vi "test-worker mode.vi"(8 "error in (no error)":errorcluster, 11 "TestCase in":refnum<class "testcase-CSMAttributes.lvclass">) -> (0 "error out":errorcluster, 3 "TestCase out":refnum<class "testcase-CSMAttributes.lvclass">)   [LabVIEW 2017, in "testcase-CSMAttributes.lvclass"]
uses:
  testcase-CSMAttributes.lvclass
  6faf3dd6-bbe3-43e6-ac0e-6a595a4bbb73.vi
  eea55257-98dc-4069-a2fc-7f3abec53d34.vi
  654a1434-e049-45b7-bbe1-b3daff27deed.vi
  232dea5e-886f-41b8-bb39-dacd9565842e.vi
  d39486ea-fbfe-4c2b-b0ae-85d31efdfc25.vi
  4fbfc3b2-4ab6-4b17-950e-362f3a1418f9.vi
  eb53d3db-f5cc-4d50-900d-3a282fe3921b.vi
  d3eb8ef0-7d19-473b-ace2-fe9805f10b86.vi
  src/user.lib/_NEVSTOP/Communicable State Machine(CSM)/AdvanceAPI/CSM - Set Module Attribute.vi
  src/user.lib/_NEVSTOP/Communicable State Machine(CSM)/AdvanceAPI/CSM - Get Module Attribute.vi
  src/user.lib/_NEVSTOP/Communicable State Machine(CSM)/Communicable State Machine.lvlib
  <vilib>/addons/_JKI Toolkits/VI Tester/TestCase.llb/TestCase.lvclass
  C:/Program Files (x86)/National Instruments/LabVIEW 2017/vi.lib/addons/_JKI Toolkits/VI Tester/TestCase.llb/TestCase.lvclass
panel:
  out "error out":errorcluster
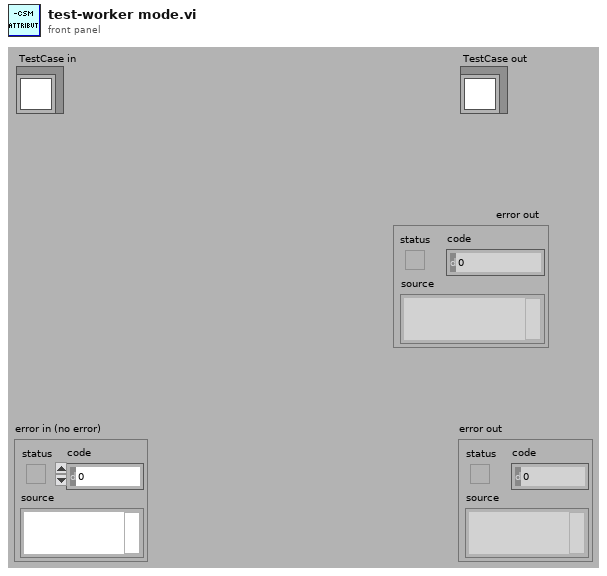
[diagram p1: front panel]
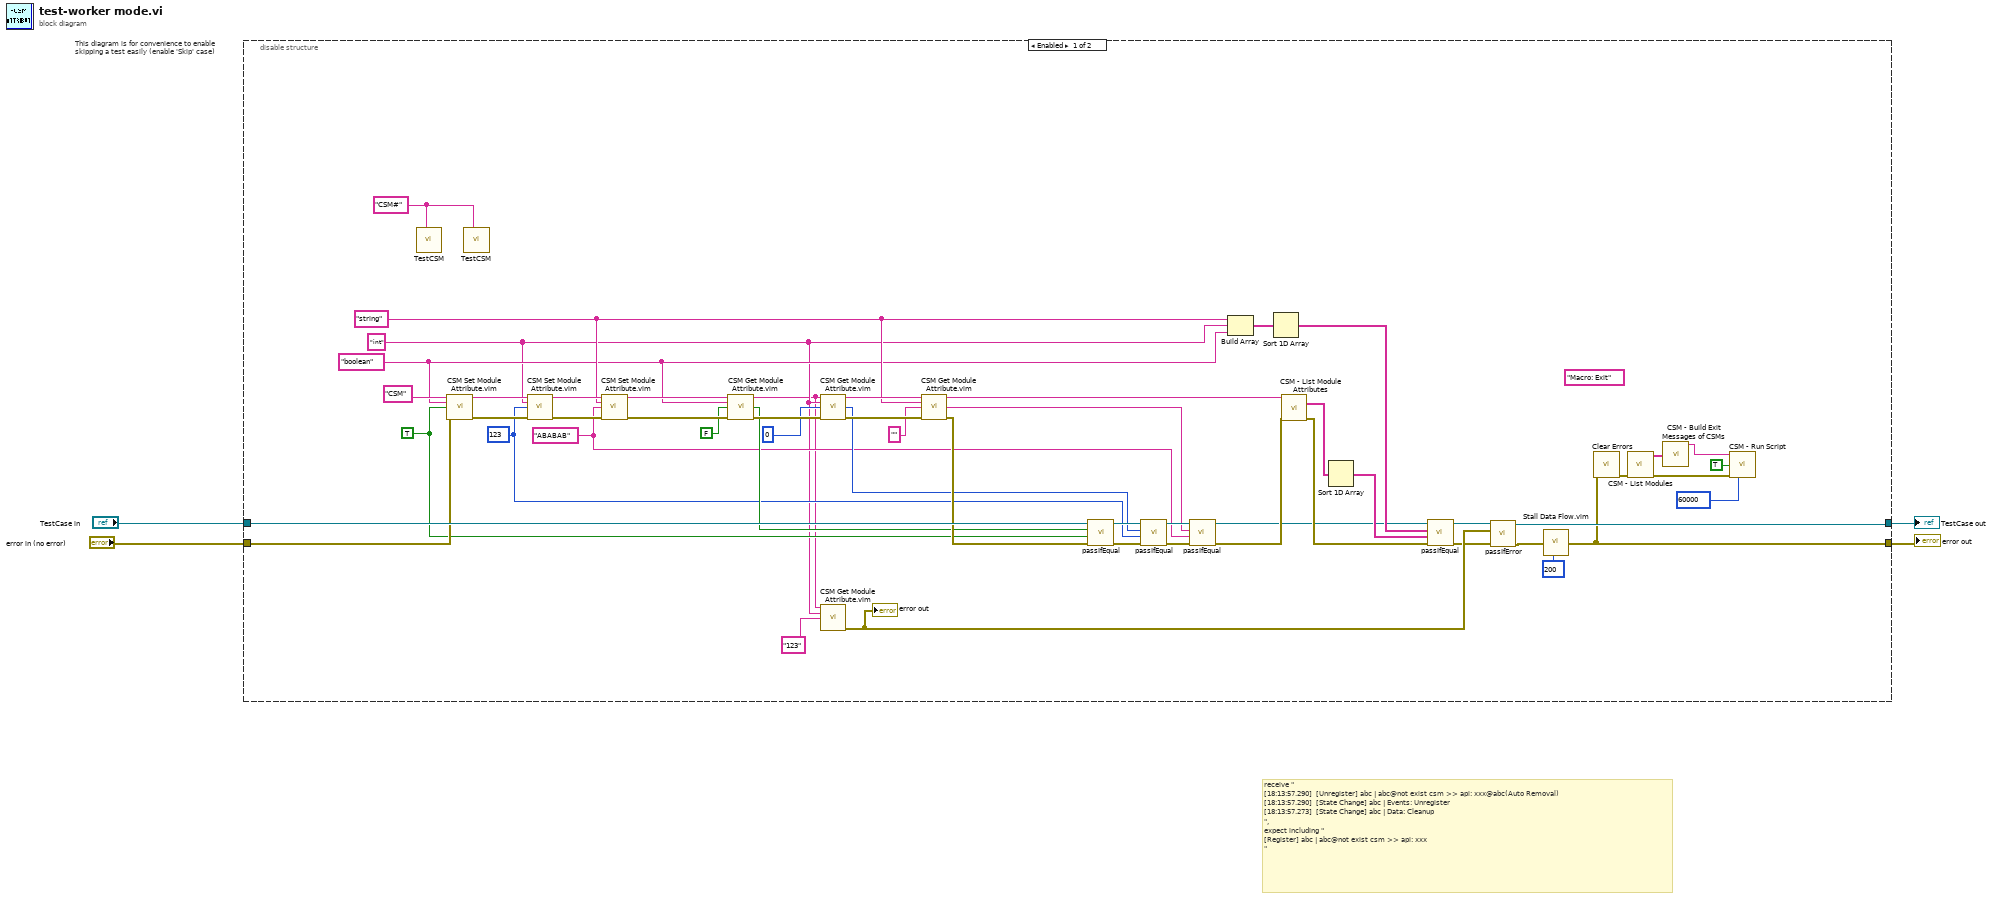
[diagram p0: block diagram]
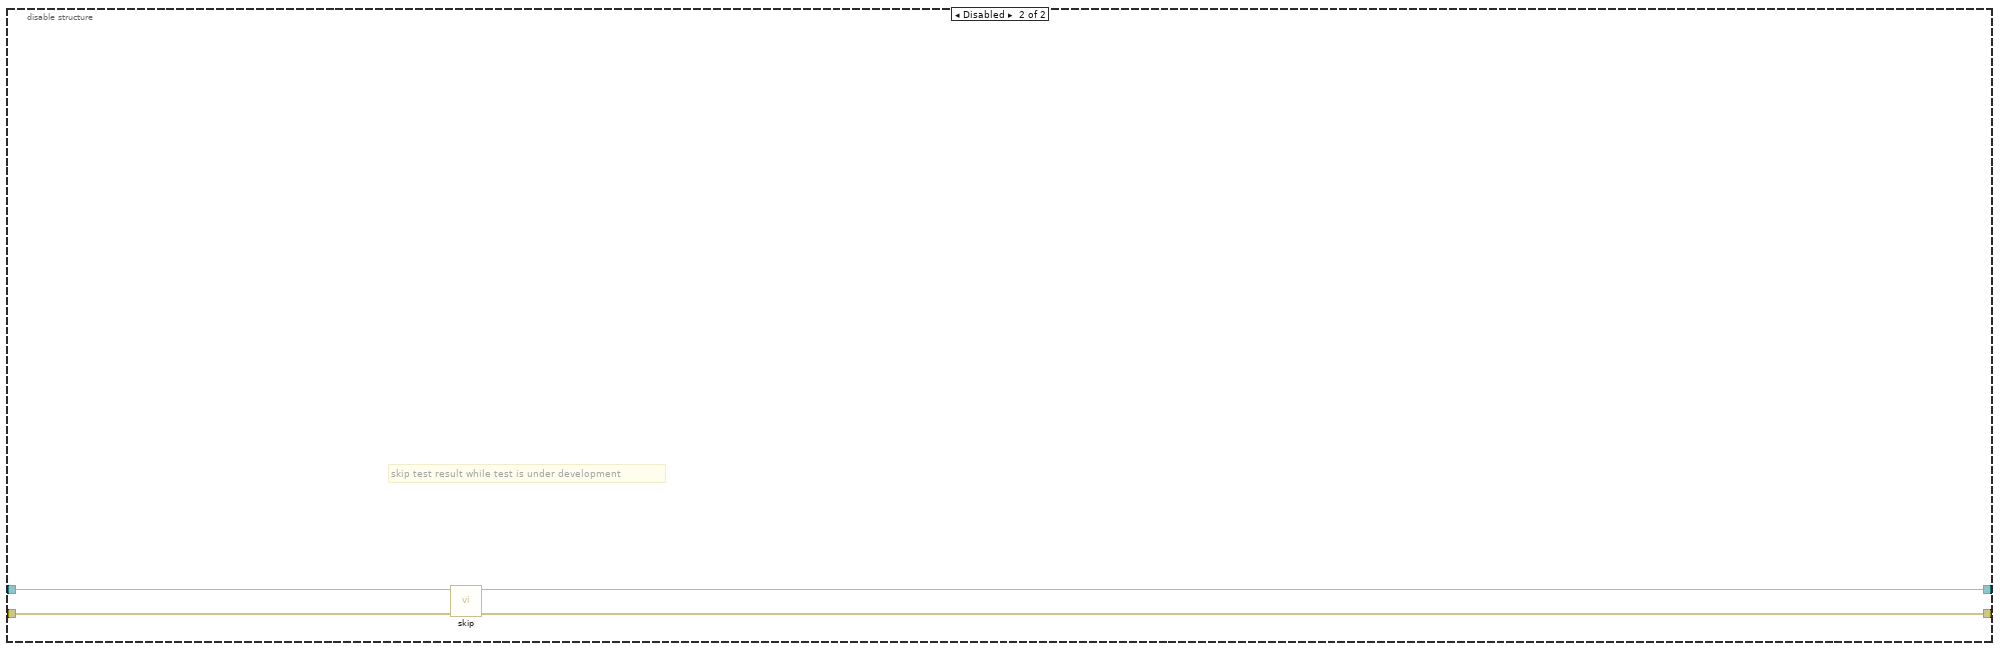
[diagram p2: hidden frame]
diagram:
  # "receive \"\n[18:13:57.290]  [Unregister] abc | abc@not exist csm >> api: xxx@abc(Auto Removal)\n[18:13:57.290]  [State Change] abc | Events: Unregister\n[18:13:57.273]  [State Change] abc | Data: Cleanup\n\", \nexpect including \"\n[Register] abc | abc@not exist csm >> api: xxx\n\""
  n1 = disable-structure "This diagram is for convenience to enable skipping a test easily (enable 'Skip' case)" shown="Enabled" {
    disable-tunnel: "TestCase in" -> [w57 w61]
    disable-tunnel: [w13 w59] -> w1
    disable-tunnel: [w7 w60] -> w3
    disable-tunnel: "error in (no error)" -> [w56 w58]
    frame Enabled {
      (unwired) "Macro: Exit" ("State")
      w32 = "ABABAB" ("Attribute")
      w28 = "string" ("Attribute")
      w36 = 123
      w19 = "int" ("Attribute")
      w41 = TRUE
      w27 = "boolean" ("Attribute")
      w12 = "CSM#" ("Name (\"\" to Use UUID)")
      n2 = call "TestCSM.vi"("Name (\"\" to Use UUID)"=w12) -> ()  [unwired: 11 in]
      n3 = call "CSM Set Module Attribute.vim"("CSM Name"="CSM" ("Name (\"\" to Use UUID)"), "Attribute"=w27, "Value"=w41, "Error In"=w56) -> ("CSM Name (Dup)"=w52:string, "error out"=w54:errorcluster)  [unwired: 8 in, 2 out]
      n4 = call "TestCSM.vi"("Name (\"\" to Use UUID)"=w12) -> ()  [unwired: 11 in]
      n5 = call "CSM Set Module Attribute.vim"("CSM Name"=w52, "Attribute"=w19, "Value"=w36, "Error In"=w54) -> ("CSM Name (Dup)"=w51:string, "error out"=w53:errorcluster)  [unwired: 8 in, 2 out]
      n6 = call "CSM Set Module Attribute.vim"("CSM Name"=w51, "Attribute"=w28, "Value"=w32, "Error In"=w53) -> ("CSM Name (Dup)"=w49:string, "error out"=w50:errorcluster)  [unwired: 8 in, 2 out]
      n7 = call "CSM Get Module Attribute.vim"("CSM Name"=w49, "Attribute"=w27, "Default Value (Empty Variant)"=FALSE, "Error In"=w50) -> ("CSM Name (Dup)"=w18:string, "Value"=w40:bool, "error out"=w48:errorcluster)  [unwired: 7 in, 2 out]
      n8 = call "CSM Get Module Attribute.vim"("CSM Name"=w18, "Attribute"=w19, "Default Value (Empty Variant)"=0, "Error In"=w48) -> ("CSM Name (Dup)"=w47:string, "Value"=w37:i32, "error out"=w46:errorcluster)  [unwired: 7 in, 2 out]
      n9 = call "CSM Get Module Attribute.vim"("CSM Name"=w18, "Attribute"=w19, "Default Value (Empty Variant)"="123") -> ("error out"=w16:errorcluster)  [unwired: 8 in, 4 out]
      "error out" <- w16
      n10 = call "CSM Get Module Attribute.vim"("CSM Name"=w47, "Attribute"=w28, "Default Value (Empty Variant)"="" ("Attribute"), "Error In"=w46) -> ("CSM Name (Dup)"=w31:string, "Value"=w33:string, "error out"=w42:errorcluster)  [unwired: 7 in, 2 out]
      n11 = call-dynamic "passIfEqual.vi"("error in (no error)"=w42, "y"=w41, "x"=w40, "TestCase in"=w57) -> ("error out"=w38:errorcluster, "TestCase out"=w39:refnum<class "testcase-CSMAttributes.lvclass">)  [unwired: 6 in]
      n12 = call-dynamic "passIfEqual.vi"("error in (no error)"=w38, "y"=w36, "x"=w37, "TestCase in"=w39) -> ("error out"=w34:errorcluster, "TestCase out"=w35:refnum<class "testcase-CSMAttributes.lvclass">)  [unwired: 6 in]
      n13 = call-dynamic "passIfEqual.vi"("error in (no error)"=w34, "y"=w32, "x"=w33, "TestCase in"=w35) -> ("error out"=w30:errorcluster, "TestCase out"=w22:refnum<class "testcase-CSMAttributes.lvclass">)  [unwired: 6 in]
      n14 = Build Array(w28, w19, w27) -> (w26:string[])
      n15 = Sort 1D Array(array=w26) -> (sorted array=w23:string[])
      n16 = call "CSM - List Module Attributes.vi"("CSM Name"=w31, "Error In"=w30) -> ("Attributes"=w25:string[], "error out"=w29:errorcluster)  [unwired: 9 in, 3 out]
      n17 = Sort 1D Array(array=w25) -> (sorted array=w24:string[])
      n18 = call-dynamic "passIfEqual.vi"("error in (no error)"=w29, "y"=w24, "x"=w23, "TestCase in"=w22) -> ("error out"=w15:errorcluster, "TestCase out"=w17:refnum<class "testcase-CSMAttributes.lvclass">)  [unwired: 6 in]
      n19 = call-dynamic "passIfError.vi"("error in (no error)"=w15, "error"=w16, "TestCase in"=w17) -> ("error out"=w14:errorcluster, "TestCase out"=w13:refnum<class "testcase-CSMAttributes.lvclass">)  [unwired: 7 in]
      n20 = call "Stall Data Flow.vim"("value in"=w14, "milliseconds to wait"=u32 200) -> ("value out"=w7:errorcluster)  [unwired: 1 out]
      n21 = call <vilib>:"Clear Errors.vi"("error in (no error)"=w7) -> ("error out"=w21:errorcluster)  [unwired: 5 in, 1 out]
      n22 = call "CSM - List Modules.vi"("Error In"=w21) -> ("error out"=w11:errorcluster, "Module Names"=w10:string[])  [unwired: 9 in]
      n23 = call "CSM - Build Exit Messages of CSMs.vi"("CSMs"=w10) -> ("States"=w8:string)  [unwired: 14 in]
      n24 = call "CSM - Run Script.vi"("CSM Scripts"=w8, "Continue If Error? (F)"=TRUE ("Continue If Error?(F)"), "error in (no error)"=w11, "Response Timeout (-2 Using Global Settings)"=60000) -> ()  [unwired: 9 in, 3 out]
    }
    frame Disabled {
      # "skip test result while test is under development"
      n25 = call <vilib>:"skip.vi"("error in (no error)"=w58, "TestCase in"=w61) -> ("error out"=w60:errorcluster, "TestCase out"=w59:refnum<class "testcase-CSMAttributes.lvclass">)  [unwired: 8 in]
    }
  }
  "error out" <- w3
  "TestCase out" <- w1
